vi "GetStatusRegisterFormat.vi"(8 "Error In":errorcluster, 11 "Keithley 6485 In":refnum<visa-resource-name>) -> (0 "Error Out":errorcluster, 2 "Status Register Format":T1, 3 "Keithley 6485 Out":refnum<visa-resource-name>)   [LabVIEW 2012, in "Keithley-6485.lvlib"]
uses:
  Keithley-6485.lvlib
  Controls/StatusRegisterFormat.ctl
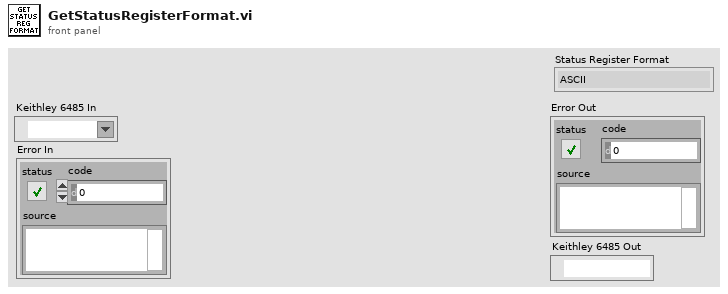
[diagram p1: front panel]
types:
  T1 = typedef "Keithley-6485.lvlib/StatusRegisterFormat.ctl" = enum16{"ASCII", "Hexadecimal", "Octal", "Binary"}
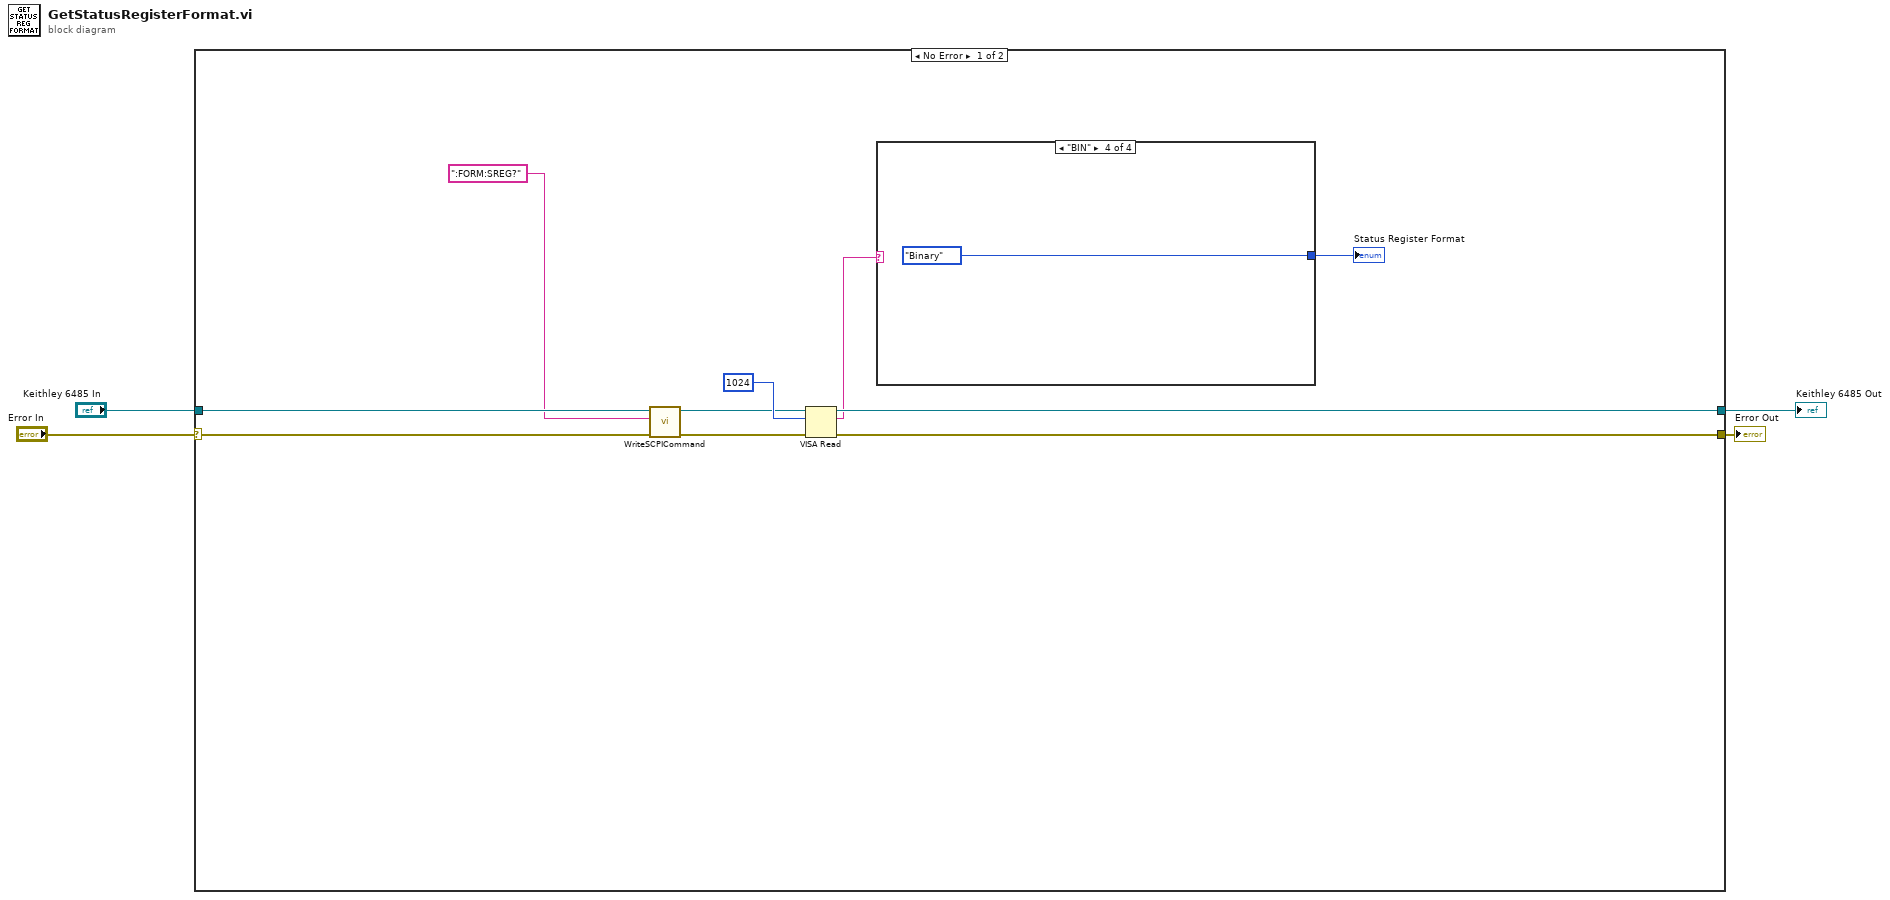
[diagram p0: block diagram]
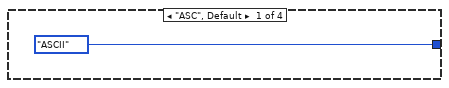
[diagram p2: hidden frame]
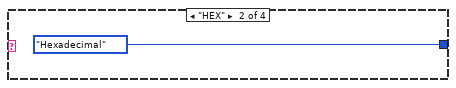
[diagram p3: hidden frame]
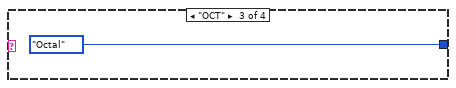
[diagram p4: hidden frame]
diagram:
  n1 = case shown="No Error" "Error In" {
    selector: "Error In" -> [w7 w19]
    tunnel: "Keithley 6485 In" -> [w6 w20]
    tunnel: [w14 w19] -> w2
    tunnel: [w13 w20] -> w1
    frame No Error {
      n2 = call "WriteSCPICommand.vi"("Error In"=w7, "SCPI Command"=":FORM:SREG?", "Keithley 6482 In"=w6) -> ("Error Out"=w8:errorcluster, "Keithley 6482 Out"=w9:refnum<visa-resource-name>)  [unwired: 7 in]
      n3 = VISA Read(VISA resource name=w9, byte count=u32 1024, error in (no error)=w8) -> (VISA resource name out=w13:refnum<visa-resource-name>, read buffer=w11:string, error out=w14:errorcluster)  [unwired: 1 out]
      n4 = case shown="\"BIN\"" w11 {
        tunnel: [StatusRegisterFormat."ASCII" ("Status Register Format") StatusRegisterFormat."Hexadecimal" ("Status Register Format") StatusRegisterFormat."Octal" ("Status Register Format") StatusRegisterFormat."Binary" ("Status Register Format")] -> w10
        frame "ASC", Default {
        }
        frame "HEX" {
        }
        frame "OCT" {
        }
        frame "BIN" {
        }
      }
      "Status Register Format" <- w10
    }
    frame Error {
    }
  }
  "Error Out" <- w2
  "Keithley 6485 Out" <- w1
